vi "Write Line.vi"(8 "error in (no error)":errorcluster, 10 "Line":string) -> (0 "error out":errorcluster)   [LabVIEW 2020, in "MGI-Console.lvlib" / "Console.lvclass"]
doc: "Writes a line to the console.\n----\nCopyright: MGI 2018\nAuthor: Derek Trepanier"
uses:
  Console.lvclass
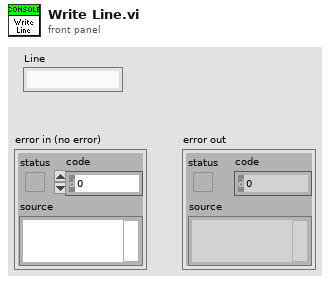
[diagram p1: front panel]
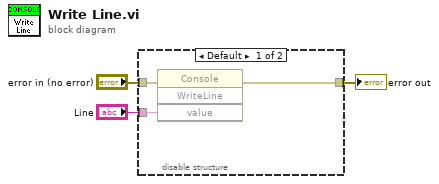
[diagram p0: block diagram]
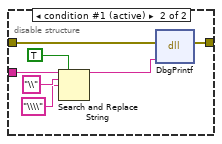
[diagram p2: hidden frame]
diagram:
  n1 = disable-structure shown="Default" {
    disable-tunnel: "error in (no error)" -> [w6 w13]
    disable-tunnel: [w5 w12] -> w2
    disable-tunnel: "Line" -> [w4 w11]
    frame condition #0 {
      n2 = invoke class="Console" method="WriteLine"(error in=w6, "value"=w4) -> (error out=w5:errorcluster)  [unwired: 2 in, 3 out]
    }
    frame condition #1 (active) {
      n3 = Search and Replace String(replace all?=TRUE ("replace all? (F)"), input string=w11, search string="\\", replace string="\\\\" ("search string")) -> (result string=w10:string)  [unwired: 4 in, 3 out]
      n4 = dll-call lib="LabVIEW" fn="DbgPrintf"(error in=w13, "arg1"=w10) -> (error out=w12:errorcluster)  [unwired: 4 in, 1 out]
    }
  }
  "error out" <- w2
